vi "GeoData.vi"() -> ()   [LabVIEW 2017] (continued)
VA\tMecklenburg County\tH1\n23915\t51117\tBaskerville\tVA\tMecklenburg County\tH1\n23071\t51119\tHartfield\tVA\tMiddlesex County\tH1\n23169\t51119\tTopping\tVA\tMiddlesex County\tH1\n23070\t51119\tHardyville\tVA\tMiddlesex County\tH1\n23175\t51119\tUrbanna\tVA\tMiddlesex County\tH1\n23176\t51119\tWake\tVA\tMiddlesex County\tH1\n23079\t51119\tJamaica\tVA\tMiddlesex County\tH1\n23031\t51119\tChristchurch\tVA\tMiddlesex County\tH1\n23092\t51119\tLocust hill\tVA\tMiddlesex County\tH1\n23032\t51119\tChurch view\tVA\tMiddlesex County\tH1\n23180\t51119\tWater view\tVA\tMiddlesex County\tH1\n22504\t51119\tLaneview\tVA\tMiddlesex County\tH1\n23043\t51119\tDeltaville\tVA\tMiddlesex County\tH1\n23149\t51119\tSaluda\tVA\tMiddlesex County\tH1\n24068\t51121\tChristiansburg\tVA\tMontgomery County\tH1\n24128\t51121\tNewport\tVA\tMontgomery County\tH1\n24061\t51121\tBlacksburg\tVA\tMontgomery County\tH1\n24063\t51121\tBlacksburg\tVA\tMontgomery County\tH1\n24149\t51121\tRiner\tVA\tMontgomery County\tH1\n24059\t51121\tBent mountain\tVA\tMontgomery County\tH1\n24347\t51121\tHiwassee\tVA\tMontgomery County\tH1\n24111\t51121\tMc coy\tVA\tMontgomery County\tH1\n24087\t51121\tElliston\tVA\tMontgomery County\tH1\n24141\t51121\tRadford\tVA\tMontgomery County\tH1\n24162\t51121\tShawsville\tVA\tMontgomery County\tH1\n24073\t51121\tChristiansburg\tVA\tMontgomery County\tH1\n24070\t51121\tCatawba\tVA\tMontgomery County\tH1\n24062\t51121\tBlacksburg\tVA\tMontgomery County\tH1\n24138\t51121\tPilot\tVA\tMontgomery County\tH1\n24060\t51121\tBlacksburg\tVA\tMontgomery County\tH1\n22920\t51125\tAfton\tVA\tNelson County\tH1\n22938\t51125\tFaber\tVA\tNelson County\tH1\n22967\t51125\tRoseland\tVA\tNelson County\tH1\n22964\t51125\tPiney river\tVA\tNelson County\tH1\n24599\t51125\tWingina\tVA\tNelson County\tH1\n22976\t51125\tTyro\tVA\tNelson County\tH1\n24483\t51125\tVesuvius\tVA\tNelson County\tH1\n22922\t51125\tArrington\tVA\tNelson County\tH1\n22949\t51125\tLovingston\tVA\tNelson County\tH1\n22952\t51125\tLyndhurst\tVA\tNelson County\tH1\n24521\t51125\tAmherst\tVA\tNelson County\tH1\n22971\t51125\tShipman\tVA\tNelson County\tH1\n24562\t51125\tHowardsville\tVA\tNelson County\tH1\n24464\t51125\tMontebello\tVA\tNelson County\tH1\n22958\t51125\tNellysford\tVA\tNelson County\tH1\n24581\t51125\tNorwood\tVA\tNelson County\tH1\n22937\t51125\tEsmont\tVA\tNelson County\tH1\n22969\t51125\tSchuyler\tVA\tNelson County\tH1\n24553\t51125\tGladstone\tVA\tNelson County\tH1\n23140\t51127\tProvidence forge\tVA\tNew Kent County\tH1\n23141\t51127\tQuinton\tVA\tNew Kent County\tH1\n23124\t51127\tNew kent\tVA\tNew Kent County\tH1\n23011\t51127\tBarhamsville\tVA\tNew Kent County\tH1\n23089\t51127\tLanexa\tVA\tNew Kent County\tH1\n23111\t51127\tMechanicsville\tVA\tNew Kent County\tH1\n23181\t51127\tWest point\tVA\tNew Kent County\tH1\n23307\t51131\tBirdsnest\tVA\tNorthampton County\tH1\n23347\t51131\tEastville\tVA\tNorthampton County\tH1\n23316\t51131\tCheriton\tVA\tNorthampton County\tH1\n23354\t51131\tFranktown\tVA\tNorthampton County\tH1\n23350\t51131\tExmore\tVA\tNorthampton County\tH1\n23413\t51131\tNassawadox\tVA\tNorthampton County\tH1\n23429\t51131\tSeaview\tVA\tNorthampton County\tH1\n23443\t51131\tTownsend\tVA\tNorthampton County\tH1\n23408\t51131\tMarionville\tVA\tNorthampton County\tH1\n23313\t51131\tCapeville\tVA\tNorthampton County\tH1\n23405\t51131\tMachipongo\tVA\tNorthampton County\tH1\n23310\t51131\tCape charles\tVA\tNorthampton County\tH1\n23398\t51131\tJamesville\tVA\tNorthampton County\tH1\n23486\t51131\tWillis wharf\tVA\tNorthampton County\tH1\n22460\t51133\tFarnham\tVA\tNorthumberland County\tH1\n22435\t51133\tCallao\tVA\tNorthumberland County\tH1\n22482\t51133\tKilmarnock\tVA\tNorthumberland County\tH1\n22503\t51133\tLancaster\tVA\tNorthumberland County\tH1\n22511\t51133\tLottsburg\tVA\tNorthumberland County\tH1\n22432\t51133\tBurgess\tVA\tNorthumberland County\tH1\n22530\t51133\tOphelia\tVA\tNorthumberland County\tH1\n22579\t51133\tWicomico church\tVA\tNorthumberland County\tH1\n22473\t51133\tHeathsville\tVA\tNorthumberland County\tH1\n22539\t51133\tReedville\tVA\tNorthumberland County\tH1\n23083\t51135\tJetersville\tVA\tNottoway County\tH1\n23922\t51135\tBurkeville\tVA\tNottoway County\tH1\n23966\t51135\tRice\tVA\tNottoway County\tH1\n23002\t51135\tAmelia court house\tVA\tNottoway County\tH1\n23955\t51135\tNottoway\tVA\tNottoway County\tH1\n23824\t51135\tBlackstone\tVA\tNottoway County\tH1\n23894\t51135\tWilsons\tVA\tNottoway County\tH1\n23930\t51135\tCrewe\tVA\tNottoway County\tH1\n23093\t51137\tLouisa\tVA\tOrange County\tH1\n22957\t51137\tMontpelier station\tVA\tOrange County\tH1\n22567\t51137\tUnionville\tVA\tOrange County\tH1\n22551\t51137\tSpotsylvania\tVA\tOrange County\tH1\n22942\t51137\tGordonsville\tVA\tOrange County\tH1\n22972\t51137\tSomerset\tVA\tOrange County\tH1\n22733\t51137\tRapidan\tVA\tOrange County\tH1\n22508\t51137\tLocust grove\tVA\tOrange County\tH1\n22923\t51137\tBarboursville\tVA\tOrange County\tH1\n22701\t51137\tCulpeper\tVA\tOrange County\tH1\n22968\t51137\tRuckersville\tVA\tOrange County\tH1\n22433\t51137\tBurr hill\tVA\tOrange County\tH1\n22542\t51137\tRhoadesville\tVA\tOrange County\tH1\n22960\t51137\tOrange\tVA\tOrange County\tH1\n22827\t51139\tElkton\tVA\tPage County\tH1\n22851\t51139\tStanley\tVA\tPage County\tH1\n22849\t51139\tShenandoah\tVA\tPage County\tH1\n22743\t51139\tSyria\tVA\tPage County\tH1\n22835\t51139\tLuray\tVA\tPage County\tH1\n22650\t51139\tRileyville\tVA\tPage County\tH1\n24133\t51141\tPatrick springs\tVA\tPatrick County\tH1\n24055\t51141\tBassett\tVA\tPatrick County\tH1\n24091\t51141\tFloyd\tVA\tPatrick County\tH1\n24317\t51141\tCana\tVA\tPatrick County\tH1\n24328\t51141\tFancy gap\tVA\tPatrick County\tH1\n24185\t51141\tWoolwine\tVA\tPatrick County\tH1\n24053\t51141\tArarat\tVA\tPatrick County\tH1\n24088\t51141\tFerrum\tVA\tPatrick County\tH1\n24165\t51141\tSpencer\tVA\tPatrick County\tH1\n24343\t51141\tHillsville\tVA\tPatrick County\tH1\n24120\t51141\tMeadows of dan\tVA\tPatrick County\tH1\n24171\t51141\tStuart\tVA\tPatrick County\tH1\n24177\t51141\tVesta\tVA\tPatrick County\tH1\n24076\t51141\tClaudville\tVA\tPatrick County\tH1\n24082\t51141\tCritz\tVA\tPatrick County\tH1\n24380\t51141\tWillis\tVA\tPatrick County\tH1\n24069\t51143\tCascade\tVA\tPittsylvania County\tH1\n24566\t51143\tKeeling\tVA\tPittsylvania County\tH1\n24565\t51143\tJava\tVA\tPittsylvania County\tH1\n24594\t51143\tSutherlin\tVA\tPittsylvania County\tH1\n24139\t51143\tPittsville\tVA\tPittsylvania County\tH1\n24540\t51143\tDanville\tVA\tPittsylvania County\tH1\n24577\t51143\tNathalie\tVA\tPittsylvania County\tH1\n24586\t51143\tRinggold\tVA\tPittsylvania County\tH1\n24054\t51143\tAxton\tVA\tPittsylvania County\tH1\n24527\t51143\tBlairs\tVA\tPittsylvania County\tH1\n24597\t51143\tVernon hill\tVA\tPittsylvania County\tH1\n24563\t51143\tHurt\tVA\tPittsylvania County\tH1\n24161\t51143\tSandy level\tVA\tPittsylvania County\tH1\n24137\t51143\tPenhook\tVA\tPittsylvania County\tH1\n24530\t51143\tCallands\tVA\tPittsylvania County\tH1\n24557\t51143\tGretna\tVA\tPittsylvania County\tH1\n24569\t51143\tLong island\tVA\tPittsylvania County\tH1\n24592\t51143\tSouth boston\tVA\tPittsylvania County\tH1\n24531\t51143\tChatham\tVA\tPittsylvania County\tH1\n24541\t51143\tDanville\tVA\tPittsylvania County\tH1\n24549\t51143\tDry fork\tVA\tPittsylvania County\tH1\n23113\t51145\tMidlothian\tVA\tPowhatan County\tH1\n23112\t51145\tMidlothian\tVA\tPowhatan County\tH1\n23160\t51145\tState farm\tVA\tPowhatan County\tH1\n23120\t51145\tMoseley\tVA\tPowhatan County\tH1\n23139\t51145\tPowhatan\tVA\tPowhatan County\tH1\n23922\t51147\tBurkeville\tVA\tPrince Edward County\tH1\n23966\t51147\tRice\tVA\tPrince Edward County\tH1\n23901\t51147\tFarmville\tVA\tPrince Edward County\tH1\n23947\t51147\tKeysville\tVA\tPrince Edward County\tH1\n23960\t51147\tProspect\tVA\tPrince Edward County\tH1\n23909\t51147\tFarmville\tVA\tPrince Edward County\tH1\n23942\t51147\tGreen bay\tVA\tPrince Edward County\tH1\n23934\t51147\tCullen\tVA\tPrince Edward County\tH1\n23954\t51147\tMeherrin\tVA\tPrince Edward County\tH1\n23943\t51147\tHampden sydney\tVA\tPrince Edward County\tH1\n23923\t51147\tCharlotte court house\tVA\tPrince Edward County\tH1\n23958\t51147\tPamplin\tVA\tPrince Edward County\tH1\n23803\t51149\tPetersburg\tVA\tPrince George County\tH1\n23842\t51149\tDisputanta\tVA\tPrince George County\tH1\n23805\t51149\tPetersburg\tVA\tPrince George County\tH1\n23860\t51149\tHopewell\tVA\tPrince George County\tH1\n23875\t51149\tPrince george\tVA\tPrince George County\tH1\n23881\t51149\tSpring grove\tVA\tPrince George County\tH1\n23801\t51149\tFort lee\tVA\tPrince George County\tH1\n23830\t51149\tCarson\tVA\tPrince George County\tH1\n20155\t51153\tGainesville\tVA\tPrince William County\tH1\n22193\t51153\tWoodbridge\tVA\tPrince William County\tH1\n20109\t51153\tManassas\tVA\tPrince William County\tH1\n20168\t51153\tHaymarket\tVA\tPrince William County\tH1\n20181\t51153\tNokesville\tVA\tPrince William County\tH1\n22026\t51153\tDumfries\tVA\tPrince William County\tH1\n22194\t51153\tWoodbridge\tVA\tPrince William County\tH1\n22192\t51153\tWoodbridge\tVA\tPrince William County\tH1\n20182\t51153\tNokesville\tVA\tPrince William County\tH1\n20111\t51153\tManassas\tVA\tPrince William County\tH1\n20110\t51153\tManassas\tVA\tPrince William County\tH1\n20137\t51153\tBroad run\tVA\tPrince William County\tH1\n22195\t51153\tWoodbridge\tVA\tPrince William County\tH1\n20112\t51153\tManassas\tVA\tPrince William County\tH1\n20169\t51153\tHaymarket\tVA\tPrince William County\tH1\n22025\t51153\tDumfries\tVA\tPrince William County\tH1\n22125\t51153\tOccoquan\tVA\tPrince William County\tH1\n22172\t51153\tTriangle\tVA\tPrince William County\tH1\n22191\t51153\tWoodbridge\tVA\tPrince William County\tH1\n20119\t51153\tCatlett\tVA\tPrince William County\tH1\n20136\t51153\tBristow\tVA\tPrince William County\tH1\n20156\t51153\tGainesville\tVA\tPrince William County\tH1\n22134\t51153\tQuantico\tVA\tPrince William County\tH1\n20143\t51153\tCatharpin\tVA\tPrince William County\tH1\n24084\t51155\tDublin\tVA\tPulaski County\tH1\n24324\t51155\tDraper\tVA\tPulaski County\tH1\n24126\t51155\tNewbern\tVA\tPulaski County\tH1\n24301\t51155\tPulaski\tVA\tPulaski County\tH1\n24347\t51155\tHiwassee\tVA\tPulaski County\tH1\n24141\t51155\tRadford\tVA\tPulaski County\tH1\n24313\t51155\tBarren springs\tVA\tPulaski County\tH1\n24058\t51155\tBelspring\tVA\tPulaski County\tH1\n22630\t51157\tFront royal\tVA\tRappahannock County\tH1\n22640\t51157\tHuntly\tVA\tRappahannock County\tH1\n22747\t51157\tWashington\tVA\tRappahannock County\tH1\n20106\t51157\tAmissville\tVA\tRappahannock County\tH1\n22716\t51157\tCastleton\tVA\tRappahannock County\tH1\n22713\t51157\tBoston\tVA\tRappahannock County\tH1\n22623\t51157\tChester gap\tVA\tRappahannock County\tH1\n22740\t51157\tSperryville\tVA\tRappahannock County\tH1\n22627\t51157\tFlint hill\tVA\tRappahannock County\tH1\n22749\t51157\tWoodville\tVA\tRappahannock County\tH1\n22460\t51159\tFarnham\tVA\tRichmond County\tH1\n22572\t51159\tWarsaw\tVA\tRichmond County\tH1\n22548\t51159\tSharps\tVA\tRichmond County\tH1\n22472\t51159\tHaynesville\tVA\tRichmond County\tH1\n22435\t51159\tCallao\tVA\tRichmond County\tH1\n22503\t51159\tLancaster\tVA\tRichmond County\tH1\n22473\t51159\tHeathsville\tVA\tRichmond County\tH1\n22520\t51159\tMontross\tVA\tRichmond County\tH1\n24014\t51161\tRoanoke\tVA\tRoanoke County\tH1\n24012\t51161\tRoanoke\tVA\tRoanoke County\tH1\n24175\t51161\tTroutville\tVA\tRoanoke County\tH1\n24065\t51161\tBoones mill\tVA\tRoanoke County\tH1\n24153\t51161\tSalem\tVA\tRoanoke County\tH1\n24059\t51161\tBent mountain\tVA\tRoanoke County\tH1\n24079\t51161\tCopper hill\tVA\tRoanoke County\tH1\n24101\t51161\tHardy\tVA\tRoanoke County\tH1\n24179\t51161\tVinton\tVA\tRoanoke County\tH1\n24020\t51161\tRoanoke\tVA\tRoanoke County\tH1\n24087\t51161\tElliston\tVA\tRoanoke County\tH1\n24019\t51161\tRoanoke\tVA\tRoanoke County\tH1\n24070\t51161\tCatawba\tVA\tRoanoke County\tH1\n24018\t51161\tRoanoke\tVA\tRoanoke County\tH1\n24015\t51161\tRoanoke\tVA\tRoanoke County\tH1\n24579\t51163\tNatural bridge station\tVA\tRockbridge County\tH1\n24416\t51163\tBuena vista\tVA\tRockbridge County\tH1\n24066\t51163\tBuchanan\tVA\tRockbridge County\tH1\n24578\t51163\tNatural bridge\tVA\tRockbridge County\tH1\n24435\t51163\tFairfield\tVA\tRockbridge County\tH1\n24450\t51163\tLexington\tVA\tRockbridge County\tH1\n24483\t51163\tVesuvius\tVA\tRockbridge County\tH1\n24472\t51163\tRaphine\tVA\tRockbridge County\tH1\n24459\t51163\tMiddlebrook\tVA\tRockbridge County\tH1\n24555\t51163\tGlasgow\tVA\tRockbridge County\tH1\n24473\t51163\tRockbridge baths\tVA\tRockbridge County\tH1\n24476\t51163\tSteeles tavern\tVA\tRockbridge County\tH1\n24415\t51163\tBrownsburg\tVA\tRockbridge County\tH1\n24439\t51163\tGoshen\tVA\tRockbridge County\tH1\n22801\t51165\tHarrisonburg\tVA\tRockingham County\tH1\n22827\t51165\tElkton\tVA\tRockingham County\tH1\n22840\t51165\tMc gaheysville\tVA\tRockingham County\tH1\n22831\t51165\tHinton\tVA\tRockingham County\tH1\n24471\t51165\tPort republic\tVA\tRockingham County\tH1\n22846\t51165\tPenn laird\tVA\tRockingham County\tH1\n22848\t51165\tPleasant valley\tVA\tRockingham County\tH1\n22833\t51165\tLacey spring\tVA\tRockingham County\tH1\n22821\t51165\tDayton\tVA\tRockingham County\tH1\n22850\t51165\tSingers glen\tVA\tRockingham County\tH1\n22849\t51165\tShenandoah\tVA\tRockingham County\tH1\n22811\t51165\tBergton\tVA\tRockingham County\tH1\n22802\t51165\tHarrisonburg\tVA\tRockingham County\tH1\n22841\t51165\tMount crawford\tVA\tRockingham County\tH1\n24486\t51165\tWeyers cave\tVA\tRockingham County\tH1\n22812\t51165\tBridgewater\tVA\tRockingham County\tH1\n24441\t51165\tGrottoes\tVA\tRockingham County\tH1\n22832\t51165\tKeezletown\tVA\tRockingham County\tH1\n22815\t51165\tBroadway\tVA\tRockingham County\tH1\n22844\t51165\tNew market\tVA\tRockingham County\tH1\n22820\t51165\tCriders\tVA\tRockingham County\tH1\n22834\t51165\tLinville\tVA\tRockingham County\tH1\n22830\t51165\tFulks run\tVA\tRockingham County\tH1\n22853\t51165\tTimberville\tVA\tRockingham County\tH1\n24237\t51167\tDante\tVA\tRussell County\tH1\n24266\t51167\tLebanon\tVA\tRussell County\tH1\n24225\t51167\tCleveland\tVA\tRussell County\tH1\n24283\t51167\tSaint paul\tVA\tRussell County\tH1\n24609\t51167\tCedar bluff\tVA\tRussell County\tH1\n24639\t51167\tRaven\tVA\tRussell County\tH1\n24224\t51167\tCastlewood\tVA\tRussell County\tH1\n24280\t51167\tRosedale\tVA\tRussell County\tH1\n24271\t51167\tNickelsville\tVA\tRussell County\tH1\n24260\t51167\tHonaker\tVA\tRussell County\tH1\n24649\t51167\tSwords creek\tVA\tRussell County\tH1\n24646\t51167\tRowe\tVA\tRussell County\tH1\n24221\t51169\tBlackwater\tVA\tScott County\tH1\n24230\t51169\tCoeburn\tVA\tScott County\tH1\n24245\t51169\tDungannon\tVA\tScott County\tH1\n24250\t51169\tFort blackmore\tVA\tScott County\tH1\n24258\t51169\tHiltons\tVA\tScott County\tH1\n24290\t51169\tWeber city\tVA\tScott County\tH1\n24202\t51169\tBristol\tVA\tScott County\tH1\n24251\t51169\tGate city\tVA\tScott County\tH1\n24271\t51169\tNickelsville\tVA\tScott County\tH1\n24244\t51169\tDuffield\tVA\tScott County\tH1\n22645\t51171\tMiddletown\tVA\tShenandoah County\tH1\n22657\t51171\tStrasburg\tVA\tShenandoah County\tH1\n22626\t51171\tFishers hill\tVA\tShenandoah County\tH1\n22842\t51171\tMount jackson\tVA\tShenandoah County\tH1\n22644\t51171\tMaurertown\tVA\tShenandoah County\tH1\n22652\t51171\tFort valley\tVA\tShenandoah County\tH1\n22810\t51171\tBasye\tVA\tShenandoah County\tH1\n22845\t51171\tOrkney springs\tVA\tShenandoah County\tH1\n22664\t51171\tWoodstock\tVA\tShenandoah County\tH1\n22847\t51171\tQuicksburg\tVA\tShenandoah County\tH1\n22824\t51171\tEdinburg\tVA\tShenandoah County\tH1\n22654\t51171\tStar tannery\tVA\tShenandoah County\tH1\n22815\t51171\tBroadway\tVA\tShenandoah County\tH1\n22844\t51171\tNew market\tVA\tShenandoah County\tH1\n22660\t51171\tToms brook\tVA\tShenandoah County\tH1\n22835\t51171\tLuray\tVA\tShenandoah County\tH1\n22853\t51171\tTimberville\tVA\tShenandoah County\tH1\n22641\t51171\tStrasburg\tVA\tShenandoah County\tH1\n24311\t51173\tAtkins\tVA\tSmyth County\tH1\n24316\t51173\tBroadford\tVA\tSmyth County\tH1\n24375\t51173\tSugar grove\tVA\tSmyth County\tH1\n24651\t51173\tTazewell\tVA\tSmyth County\tH1\n24340\t51173\tGlade spring\tVA\tSmyth County\tH1\n24354\t51173\tMarion\tVA\tSmyth County\tH1\n24318\t51173\tCeres\tVA\tSmyth County\tH1\n24370\t51173\tSaltville\tVA\tSmyth County\tH1\n24368\t51173\tRural retreat\tVA\tSmyth County\tH1\n24378\t51173\tTroutdale\tVA\tSmyth County\tH1\n24236\t51173\tDamascus\tVA\tSmyth County\tH1\n24319\t51173\tChilhowie\tVA\tSmyth County\tH1\n24374\t51173\tSpeedwell\tVA\tSmyth County\tH1\n23867\t51175\tJarratt\tVA\tSouthampton County\tH1\n23878\t51175\tSedley\tVA\tSouthampton County\tH1\n23847\t51175\tEmporia\tVA\tSouthampton County\tH1\n23851\t51175\tFranklin\tVA\tSouthampton County\tH1\n23898\t51175\tZuni\tVA\tSouthampton County\tH1\n23837\t51175\tCourtland\tVA\tSouthampton County\tH1\n23844\t51175\tDrewryville\tVA\tSouthampton County\tH1\n23827\t51175\tBoykins\tVA\tSouthampton County\tH1\n23829\t51175\tCapron\tVA\tSouthampton County\tH1\n23828\t51175\tBranchville\tVA\tSouthampton County\tH1\n23866\t51175\tIvor\tVA\tSouthampton County\tH1\n23874\t51175\tNewsoms\tVA\tSouthampton County\tH1\n23888\t51175\tWakefield\tVA\tSouthampton County\tH1\n22408\t51177\tFredericksburg\tVA\tSpotsylvania County\tH1\n22553\t51177\tSpotsylvania\tVA\tSpotsylvania County\tH1\n22534\t51177\tPartlow\tVA\tSpotsylvania County\tH1\n23117\t51177\tMineral\tVA\tSpotsylvania County\tH1\n22567\t51177\tUnionville\tVA\tSpotsylvania County\tH1\n22551\t51177\tSpotsylvania\tVA\tSpotsylvania County\tH1\n22546\t51177\tRuther glen\tVA\tSpotsylvania County\tH1\n22508\t51177\tLocust grove\tVA\tSpotsylvania County\tH1\n22580\t51177\tWoodford\tVA\tSpotsylvania County\tH1\n22404\t51177\tFredericksburg\tVA\tSpotsylvania County\tH1\n23015\t51177\tBeaverdam\tVA\tSpotsylvania County\tH1\n22401\t51177\tFredericksburg\tVA\tSpotsylvania County\tH1\n22407\t51177\tFredericksburg\tVA\tSpotsylvania County\tH1\n22960\t51177\tOrange\tVA\tSpotsylvania County\tH1\n23024\t51177\tBumpass\tVA\tSpotsylvania County\tH1\n22565\t51177\tThornburg\tVA\tSpotsylvania County\tH1\n22406\t51179\tFredericksburg\tVA\tStafford County\tH1\n22405\t51179\tFredericksburg\tVA\tStafford County\tH1\n22554\t51179\tStafford\tVA\tStafford County\tH1\n22545\t51179\tRuby\tVA\tStafford County\tH1\n22412\t51179\tFredericksburg\tVA\tStafford County\tH1\n22555\t51179\tStafford\tVA\tStafford County\tH1\n22135\t51179\tQuantico\tVA\tStafford County\tH1\n22556\t51179\tStafford\tVA\tStafford County\tH1\n22403\t51179\tFredericksburg\tVA\tStafford County\tH1\n22430\t51179\tBrooke\tVA\tStafford County\tH1\n22471\t51179\tHartwood\tVA\tStafford County\tH1\n22728\t51179\tMidland\tVA\tStafford County\tH1\n22463\t51179\tGarrisonville\tVA\tStafford County\tH1\n22134\t51179\tQuantico\tVA\tStafford County\tH1\n23846\t51181\tElberon\tVA\tSurry County\tH1\n23890\t51181\tWaverly\tVA\tSurry County\tH1\n23899\t51181\tClaremont\tVA\tSurry County\tH1\n23842\t51181\tDisputanta\tVA\tSurry County\tH1\n23883\t51181\tSurry\tVA\tSurry County\tH1\n23839\t51181\tDendron\tVA\tSurry County\tH1\n23430\t51181\tSmithfield\tVA\tSurry County\tH1\n23881\t51181\tSpring grove\tVA\tSurry County\tH1\n23866\t51181\tIvor\tVA\tSurry County\tH1\n23888\t51181\tWakefield\tVA\tSurry County\tH1\n23867\t51183\tJarratt\tVA\tSussex County\tH1\n23878\t51183\tSedley\tVA\tSussex County\tH1\n23890\t51183\tWaverly\tVA\tSussex County\tH1\n23847\t51183\tEmporia\tVA\tSussex County\tH1\n23842\t51183\tDisputanta\tVA\tSussex County\tH1\n23891\t51183\tWaverly\tVA\tSussex County\tH1\n23897\t51183\tYale\tVA\tSussex County\tH1\n23837\t51183\tCourtland\tVA\tSussex County\tH1\n23829\t51183\tCapron\tVA\tSussex County\tH1\n23882\t51183\tStony creek\tVA\tSussex County\tH1\n23830\t51183\tCarson\tVA\tSussex County\tH1\n23888\t51183\tWakefield\tVA\tSussex County\tH1\n23884\t51183\tSussex\tVA\tSussex County\tH1\n24630\t51185\tNorth tazewell\tVA\tTazewell County\tH1\n24316\t51185\tBroadford\tVA\tTazewell County\tH1\n24604\t51185\tBishop\tVA\tTazewell County\tH1\n24314\t51185\tBastian\tVA\tTazewell County\tH1\n24651\t51185\tTazewell\tVA\tTazewell County\tH1\n24602\t51185\tBandy\tVA\tTazewell County\tH1\n24622\t51185\tJewell ridge\tVA\tTazewell County\tH1\n24612\t51185\tDoran\tVA\tTazewell County\tH1\n24647\t51185\tShortt gap\tVA\tTazewell County\tH1\n24377\t51185\tTannersville\tVA\tTazewell County\tH1\n24609\t51185\tCedar bluff\tVA\tTazewell County\tH1\n24606\t51185\tBoissevain\tVA\tTazewell County\tH1\n24640\t51185\tRed ash\tVA\tTazewell County\tH1\n24641\t51185\tRichlands\tVA\tTazewell County\tH1\n24619\t51185\tHorsepen\tVA\tTazewell County\tH1\n24639\t51185\tRaven\tVA\tTazewell County\tH1\n24635\t51185\tPocahontas\tVA\tTazewell County\tH1\n24608\t51185\tBurkes garden\tVA\tTazewell County\tH1\n24605\t51185\tBluefield\tVA\tTazewell County\tH1\n24637\t51185\tPounding mill\tVA\tTazewell County\tH1\n24601\t51185\tAmonate\tVA\tTazewell County\tH1\n24613\t51185\tFalls mills\tVA\tTazewell County\tH1\n22630\t51187\tFront royal\tVA\tWarren County\tH1\n22645\t51187\tMiddletown\tVA\tWarren County\tH1\n22649\t51187\tMiddletown\tVA\tWarren County\tH1\n22657\t51187\tStrasburg\tVA\tWarren County\tH1\n22623\t51187\tChester gap\tVA\tWarren County\tH1\n22642\t51187\tLinden\tVA\tWarren County\tH1\n22610\t51187\tBentonville\tVA\tWarren County\tH1\n22655\t51187\tStephens city\tVA\tWarren County\tH1\n22663\t51187\tWhite post\tVA\tWarren County\tH1\n24212\t51191\tAbingdon\tVA\tWashington County\tH1\n24361\t51191\tMeadowview\tVA\tWashington County\tH1\n24327\t51191\tEmory\tVA\tWashington County\tH1\n24340\t51191\tGlade spring\tVA\tWashington County\tH1\n24258\t51191\tHiltons\tVA\tWashington County\tH1\n24370\t51191\tSaltville\tVA\tWashington County\tH1\n24211\t51191\tAbingdon\tVA\tWashington County\tH1\n24270\t51191\tMendota\tVA\tWashington County\tH1\n24202\t51191\tBristol\tVA\tWashington County\tH1\n24210\t51191\tAbingdon\tVA\tWashington County\tH1\n24292\t51191\tWhitetop\tVA\tWashington County\tH1\n24236\t51191\tDamascus\tVA\tWashington County\tH1\n24319\t51191\tChilhowie\tVA\tWashington County\tH1\n22572\t51193\tWarsaw\tVA\tWestmoreland County\tH1\n22529\t51193\tOldhams\tVA\tWestmoreland County\tH1\n22435\t51193\tCallao\tVA\tWestmoreland County\tH1\n22442\t51193\tColes point\tVA\tWestmoreland County\tH1\n22581\t51193\tZacata\tVA\tWestmoreland County\tH1\n22524\t51193\tMount holly\tVA\tWestmoreland County\tH1\n22558\t51193\tStratford\tVA\tWestmoreland County\tH1\n22443\t51193\tColonial beach\tVA\tWestmoreland County\tH1\n22469\t51193\tHague\tVA\tWestmoreland County\tH1\n22485\t51193\tKing george\tVA\tWestmoreland County\tH1\n22488\t51193\tKinsale\tVA\tWestmoreland County\tH1\n22577\t51193\tSandy point\tVA\tWestmoreland County\tH1\n22520\t51193\tMontross\tVA\tWestmoreland County\tH1\n24219\t51195\tBig stone gap\tVA\tWise County\tH1\n24230\t51195\tCoeburn\tVA\tWise County\tH1\n24283\t51195\tSaint paul\tVA\tWise County\tH1\n24293\t51195\tWise\tVA\tWise County\tH1\n24246\t51195\tEast stone gap\tVA\tWise County\tH1\n24273\t51195\tNorton\tVA\tWise County\tH1\n24279\t51195\tPound\tVA\tWise County\tH1\n24215\t51195\tAndover\tVA\tWise County\tH1\n24216\t51195\tAppalachia\tVA\tWise County\tH1\n24324\t51197\tDraper\tVA\tWythe County\tH1\n24360\t51197\tMax meadows\tVA\tWythe County\tH1\n24322\t51197\tCripple creek\tVA\tWythe County\tH1\n24350\t51197\tIvanhoe\tVA\tWythe County\tH1\n24343\t51197\tHillsville\tVA\tWythe County\tH1\n24368\t51197\tRural retreat\tVA\tWythe County\tH1\n24313\t51197\tBarren springs\tVA\tWythe County\tH1\n24312\t51197\tAustinville\tVA\tWythe County\tH1\n24382\t51197\tWytheville\tVA\tWythe County\tH1\n24323\t51197\tCrockett\tVA\tWythe County\tH1\n24374\t51197\tSpeedwell\tVA\tWythe County\tH1\n23185\t51199\tWilliamsburg\tVA\tYork County\tH1\n23602\t51199\tNewport news\tVA\tYork County\tH1\n23692\t51199\tYorktown\tVA\tYork County\tH1\n23696\t51199\tSeaford\tVA\tYork County\tH1\n23188\t51199\tWilliamsburg\tVA\tYork County\tH1\n23691\t51199\tYorktown\tVA\tYork County\tH1\n23693\t51199\tYorktown\tVA\tYork County\tH1\n23603\t51199\tNewport news\tVA\tYork County\tH1\n23690\t51199\tYorktown\tVA\tYork County\tH1\n23665\t51199\tHampton\tVA\tYork County\tH1\n23694\t51199\tLackey\tVA\tYork County\tH1\n23090\t51199\tLightfoot\tVA\tYork County\tH1\n22305\t51510\tAlexandria\tVA\tAlexandria city\tC7\n22350\t51510\tAlexandria\tVA\tAlexandria city\tC7\n22320\t51510\tAlexandria\tVA\tAlexandria city\tC7\n22312\t51510\tAlexandria\tVA\tAlexandria city\tC7\n22332\t51510\tAlexandria\tVA\tAlexandria city\tC7\n22333\t51510\tAlexandria\tVA\tAlexandria city\tC7\n22302\t51510\tAlexandria\tVA\tAlexandria city\tC7\n22304\t51510\tAlexandria\tVA\tAlexandria city\tC7\n22314\t51510\tAlexandria\tVA\tAlexandria city\tC7\n22313\t51510\tAlexandria\tVA\tAlexandria city\tC7\n20598\t51510\tDhs\tVA\tAlexandria city\tC7\n22301\t51510\tAlexandria\tVA\tAlexandria city\tC7\n22331\t51510\tAlexandria\tVA\tAlexandria city\tC7\n22206\t51510\tArlington\tVA\tAlexandria city\tC7\n22311\t51510\tAlexandria\tVA\tAlexandria city\tC7\n24203\t51520\tBristol\tVA\tBristol city\tC7\n24201\t51520\tBristol\tVA\tBristol city\tC7\n24202\t51520\tBristol\tVA\tBristol city\tC7\n24209\t51520\tBristol\tVA\tBristol city\tC7\n24416\t51530\tBuena vista\tVA\tBuena Vista city\tC7\n22903\t51540\tCharlottesville\tVA\tCharlottesville city\tC7\n22901\t51540\tCharlottesville\tVA\tCharlottesville city\tC7\n22902\t51540\tCharlottesville\tVA\tCharlottesville city\tC7\n22906\t51540\tCharlottesville\tVA\tCharlottesville city\tC7\n22908\t51540\tCharlottesville\tVA\tCharlottesville city\tC7\n22905\t51540\tCharlottesville\tVA\tCharlottesville city\tC7\n23323\t51550\tChesapeake\tVA\tChesapeake city\tC7\n23326\t51550\tChesapeake\tVA\tChesapeake city\tC7\n23322\t51550\tChesapeake\tVA\tChesapeake city\tC7\n23320\t51550\tChesapeake\tVA\tChesapeake city\tC7\n23321\t51550\tChesapeake\tVA\tChesapeake city\tC7\n23324\t51550\tChesapeake\tVA\tChesapeake city\tC7\n23703\t51550\tPortsmouth\tVA\tChesapeake city\tC7\n23328\t51550\tChesapeake\tVA\tChesapeake city\tC7\n23325\t51550\tChesapeake\tVA\tChesapeake city\tC7\n23435\t51550\tSuffolk\tVA\tChesapeake city\tC7\n23702\t51550\tPortsmouth\tVA\tChesapeake city\tC7\n23327\t51550\tChesapeake\tVA\tChesapeake city\tC7\n23464\t51550\tVirginia beach\tVA\tChesapeake city\tC7\n23834\t51570\tColonial heights\tVA\tColonial Heights city\tC7\n24426\t51580\tCovington\tVA\tCovington city\tC7\n24540\t51590\tDanville\tVA\tDanville city\tC7\n24541\t51590\tDanville\tVA\tDanville city\tC7\n23847\t51595\tEmporia\tVA\tEmporia city\tC7\n22030\t51600\tFairfax\tVA\tFairfax city\tC7\n22038\t51600\tFairfax\tVA\tFairfax city\tC7\n22031\t51600\tFairfax\tVA\tFairfax city\tC7\n22032\t51600\tFairfax\tVA\tFairfax city\tC7\n22205\t51610\tArlington\tVA\tFalls Church city\tC7\n22044\t51610\tFalls church\tVA\tFalls Church city\tC7\n22046\t51610\tFalls church\tVA\tFalls Church city\tC7\n22213\t51610\tArlington\tVA\tFalls Church city\tC7\n22042\t51610\tFalls church\tVA\tFalls Church city\tC7\n22040\t51610\tFalls church\tVA\tFalls Church city\tC7\n23851\t51620\tFranklin\tVA\tFranklin city\tC7\n22408\t51630\tFredericksburg\tVA\tFredericksburg city\tC7\n22402\t51630\tFredericksburg\tVA\tFredericksburg city\tC7\n22404\t51630\tFredericksburg\tVA\tFredericksburg city\tC7\n22401\t51630\tFredericksburg\tVA\tFredericksburg city\tC7\n22407\t51630\tFredericksburg\tVA\tFredericksburg city\tC7\n24333\t51640\tGalax\tVA\tGalax city\tC7\n23607\t51650\tNewport news\tVA\tHampton city\tC7\n23670\t51650\tHampton\tVA\tHampton city\tC7\n23663\t51650\tHampton\tVA\tHampton city\tC7\n23669\t51650\tHampton\tVA\tHampton city\tC7\n23662\t51650\tPoquoson\tVA\tHampton city\tC7\n23651\t51650\tFort monroe\tVA\tHampton city\tC7\n23666\t51650\tHampton\tVA\tHampton city\tC7\n23668\t51650\tHampton\tVA\tHampton city\tC7\n23630\t51650\tHampton\tVA\tHampton city\tC7\n23661\t51650\tHampton\tVA\tHampton city\tC7\n23665\t51650\tHampton\tVA\tHampton city\tC7\n23605\t51650\tNewport news\tVA\tHampton city\tC7\n23681\t51650\tHampton\tVA\tHampton city\tC7\n23664\t51650\tHampton\tVA\tHampton city\tC7\n23667\t51650\tHampton\tVA\tHampton city\tC7\n22801\t51660\tHarrisonburg\tVA\tHarrisonburg city\tC7\n22802\t51660\tHarrisonburg\tVA\tHarrisonburg city\tC7\n22803\t51660\tHarrisonburg\tVA\tHarrisonburg city\tC7\n22807\t51660\tHarrisonburg\tVA\tHarrisonburg city\tC7\n23860\t51670\tHopewell\tVA\tHopewell city\tC7\n24450\t51678\tLexington\tVA\tLexington city\tC7\n24515\t51680\tLynchburg\tVA\tLynchburg city\tC7\n24504\t51680\tLynchburg\tVA\tLynchburg city\tC7\n24503\t51680\tLynchburg\tVA\tLynchburg city\tC7\n24506\t51680\tLynchburg\tVA\tLynchburg city\tC7\n24513\t51680\tLynchburg\tVA\tLynchburg city\tC7\n24502\t51680\tLynchburg\tVA\tLynchburg city\tC7\n24514\t51680\tLynchburg\tVA\tLynchburg city\tC7\n24501\t51680\tLynchburg\tVA\tLynchburg city\tC7\n24551\t51680\tForest\tVA\tLynchburg city\tC7\n20110\t51683\tManassas\tVA\tManassas city\tC7\n20108\t51683\tManassas\tVA\tManassas city\tC7\n20111\t51685\tManassas\tVA\tManassas Park city\tC7\n20110\t51685\tManassas\tVA\tManassas Park city\tC7\n20113\t51685\tManassas\tVA\tManassas Park city\tC7\n24112\t51690\tMartinsville\tVA\tMartinsville city\tC7\n23606\t51700\tNewport news\tVA\tNewport News city\tC7\n23601\t51700\tNewport news\tVA\tNewport News city\tC7\n23602\t51700\tNewport news\tVA\tNewport News city\tC7\n23607\t51700\tNewport news\tVA\tNewport News city\tC7\n23609\t51700\tNewport news\tVA\tNewport News city\tC7\n23670\t51700\tHampton\tVA\tNewport News city\tC7\n23604\t51700\tFort eustis\tVA\tNewport News city\tC7\n23612\t51700\tNewport news\tVA\tNewport News city\tC7\n23608\t51700\tNewport news\tVA\tNewport News city\tC7\n23666\t51700\tHampton\tVA\tNewport News city\tC7\n23630\t51700\tHampton\tVA\tNewport News city\tC7\n23603\t51700\tNewport news\tVA\tNewport News city\tC7\n23690\t51700\tYorktown\tVA\tNewport News city\tC7\n23605\t51700\tNewport news\tVA\tNewport News city\tC7\n23628\t51700\tNewport news\tVA\tNewport News city\tC7\n23505\t51710\tNorfolk\tVA\tNorfolk city\tC7\n23510\t51710\tNorfolk\tVA\tNorfolk city\tC7\n23551\t51710\tNorfolk\tVA\tNorfolk city\tC7\n23503\t51710\tNorfolk\tVA\tNorfolk city\tC7\n23509\t51710\tNorfolk\tVA\tNorfolk city\tC7\n23513\t51710\tNorfolk\tVA\tNorfolk city\tC7\n23529\t51710\tNorfolk\tVA\tNorfolk city\tC7\n23462\t51710\tVirginia beach\tVA\tNorfolk city\tC7\n23518\t51710\tNorfolk\tVA\tNorfolk city\tC7\n23523\t51710\tNorfolk\tVA\tNorfolk city\tC7\n23502\t51710\tNorfolk\tVA\tNorfolk city\tC7\n23511\t51710\tNorfolk\tVA\tNorfolk city\tC7\n23517\t51710\tNorfolk\tVA\tNorfolk city\tC7\n23514\t51710\tNorfolk\tVA\tNorfolk city\tC7\n23504\t51710\tNorfolk\tVA\tNorfolk city\tC7\n23515\t51710\tNorfolk\tVA\tNorfolk city\tC7\n23507\t51710\tNorfolk\tVA\tNorfolk city\tC7\n23501\t51710\tNorfolk\tVA\tNorfolk city\tC7\n23541\t51710\tNorfolk\tVA\tNorfolk city\tC7\n23508\t51710\tNorfolk\tVA\tNorfolk city\tC7\n24273\t51720\tNorton\tVA\tNorton city\tC7\n23803\t51730\tPetersburg\tVA\tPetersburg city\tC7\n23805\t51730\tPetersburg\tVA\tPetersburg city\tC7\n23875\t51730\tPrince george\tVA\tPetersburg city\tC7\n23801\t51730\tFort lee\tVA\tPetersburg city\tC7\n23804\t51730\tPetersburg\tVA\tPetersburg city\tC7\n23662\t51735\tPoquoson\tVA\tPoquoson city\tC7\n23708\t51740\tPortsmouth\tVA\tPortsmouth city\tC7\n23705\t51740\tPortsmouth\tVA\tPortsmouth city\tC7\n23709\t51740\tPortsmouth\tVA\tPortsmouth city\tC7\n23321\t51740\tChesapeake\tVA\tPortsmouth city\tC7\n23704\t51740\tPortsmouth\tVA\tPortsmouth city\tC7\n23703\t51740\tPortsmouth\tVA\tPortsmouth city\tC7\n23701\t51740\tPortsmouth\tVA\tPortsmouth city\tC7\n23707\t51740\tPortsmouth\tVA\tPortsmouth city\tC7\n23702\t51740\tPortsmouth\tVA\tPortsmouth city\tC7\n24129\t51750\tNew river\tVA\tRadford city\tC7\n24141\t51750\tRadford\tVA\tRadford city\tC7\n24073\t51750\tChristiansburg\tVA\tRadford city\tC7\n24142\t51750\tRadford\tVA\tRadford city\tC7\n24132\t51750\tParrott\tVA\tRadford city\tC7\n23222\t51760\tRichmond\tVA\tRichmond city\tC7\n23221\t51760\tRichmond\tVA\tRichmond city\tC7\n23224\t51760\tRichmond\tVA\tRichmond city\tC7\n23235\t51760\tRichmond\tVA\tRichmond city\tC7\n23218\t51760\tRichmond\tVA\tRichmond city\tC7\n23249\t51760\tRichmond\tVA\tRichmond city\tC7\n23113\t51760\tMidlothian\tVA\tRichmond city\tC7\n23219\t51760\tRichmond\tVA\tRichmond city\tC7\n23231\t51760\tHenrico\tVA\tRichmond city\tC7\n23293\t51760\tRichmond\tVA\tRichmond city\tC7\n23269\t51760\tRichmond\tVA\tRichmond city\tC7\n23220\t51760\tRichmond\tVA\tRichmond city\tC7\n23284\t51760\tRichmond\tVA\tRichmond city\tC7\n23298\t51760\tRichmond\tVA\tRichmond city\tC7\n23241\t51760\tRichmond\tVA\tRichmond city\tC7\n23227\t51760\tRichmond\tVA\tRichmond city\tC7\n23260\t51760\tRichmond\tVA\tRichmond city\tC7\n23223\t51760\tRichmond\tVA\tRichmond city\tC7\n23261\t51760\tRichmond\tVA\tRichmond city\tC7\n23173\t51760\tRichmond\tVA\tRichmond city\tC7\n23226\t51760\tRichmond\tVA\tRichmond city\tC7\n23286\t51760\tRichmond\tVA\tRichmond city\tC7\n23228\t51760\tHenrico\tVA\tRichmond city\tC7\n23230\t51760\tRichmond\tVA\tRichmond city\tC7\n23234\t51760\tRichmond\tVA\tRichmond city\tC7\n23232\t51760\tRichmond\tVA\tRichmond city\tC7\n23225\t51760\tRichmond\tVA\tRichmond city\tC7\n24014\t51770\tRoanoke\tVA\tRoanoke city\tC7\n24012\t51770\tRoanoke\tVA\tRoanoke city\tC7\n24026\t51770\tRoanoke\tVA\tRoanoke city\tC7\n24035\t51770\tRoanoke\tVA\tRoanoke city\tC7\n24036\t51770\tRoanoke\tVA\tRoanoke city\tC7\n24030\t51770\tRoanoke\tVA\tRoanoke city\tC7\n24001\t51770\tRoanoke\tVA\tRoanoke city\tC7\n24042\t51770\tRoanoke\tVA\tRoanoke city\tC7\n24011\t51770\tRoanoke\tVA\tRoanoke city\tC7\n24022\t51770\tRoanoke\tVA\tRoanoke city\tC7\n24153\t51770\tSalem\tVA\tRoanoke city\tC7\n24010\t51770\tRoanoke\tVA\tRoanoke city\tC7\n24031\t51770\tRoanoke\tVA\tRoanoke city\tC7\n24009\t51770\tRoanoke\tVA\tRoanoke city\tC7\n24028\t51770\tRoanoke\tVA\tRoanoke city\tC7\n24034\t51770\tRoanoke\tVA\tRoanoke city\tC7\n24179\t51770\tVinton\tVA\tRoanoke city\tC7\n24027\t51770\tRoanoke\tVA\tRoanoke city\tC7\n24023\t51770\tRoanoke\tVA\tRoanoke city\tC7\n24013\t51770\tRoanoke\tVA\tRoanoke city\tC7\n24006\t51770\tRoanoke\tVA\tRoanoke city\tC7\n24007\t51770\tRoanoke\tVA\tRoanoke city\tC7\n24037\t51770\tRoanoke\tVA\tRoanoke city\tC7\n24016\t51770\tRoanoke\tVA\tRoanoke city\tC7\n24017\t51770\tRoanoke\tVA\tRoanoke city\tC7\n24032\t51770\tRoanoke\tVA\tRoanoke city\tC7\n24008\t51770\tRoanoke\tVA\tRoanoke city\tC7\n24003\t51770\tRoanoke\tVA\tRoanoke city\tC7\n24019\t51770\tRoanoke\tVA\tRoanoke city\tC7\n24005\t51770\tRoanoke\tVA\tRoanoke city\tC7\n24004\t51770\tRoanoke\tVA\tRoanoke city\tC7\n24025\t51770\tRoanoke\tVA\tRoanoke city\tC7\n24024\t51770\tRoanoke\tVA\tRoanoke city\tC7\n24018\t51770\tRoanoke\tVA\tRoanoke city\tC7\n24015\t51770\tRoanoke\tVA\tRoanoke city\tC7\n24038\t51770\tRoanoke\tVA\tRoanoke city\tC7\n24002\t51770\tRoanoke\tVA\tRoanoke city\tC7\n24033\t51770\tRoanoke\tVA\tRoanoke city\tC7\n24029\t51770\tRoanoke\tVA\tRoanoke city\tC7\n24153\t51775\tSalem\tVA\tSalem city\tC7\n24017\t51775\tRoanoke\tVA\tSalem city\tC7\n24019\t51775\tRoanoke\tVA\tSalem city\tC7\n24018\t51775\tRoanoke\tVA\tSalem city\tC7\n24402\t51790\tStaunton\tVA\tStaunton city\tC7\n24482\t51790\tVerona\tVA\tStaunton city\tC7\n24401\t51790\tStaunton\tVA\tStaunton city\tC7\n23432\t51800\tSuffolk\tVA\tSuffolk city\tC7\n23439\t51800\tSuffolk\tVA\tSuffolk city\tC7\n23434\t51800\tSuffolk\tVA\tSuffolk city\tC7\n23438\t51800\tSuffolk\tVA\tSuffolk city\tC7\n23321\t51800\tChesapeake\tVA\tSuffolk city\tC7\n23487\t51800\tWindsor\tVA\tSuffolk city\tC7\n23437\t51800\tSuffolk\tVA\tSuffolk city\tC7\n23430\t51800\tSmithfield\tVA\tSuffolk city\tC7\n23436\t51800\tSuffolk\tVA\tSuffolk city\tC7\n23435\t51800\tSuffolk\tVA\tSuffolk city\tC7\n23433\t51800\tSuffolk\tVA\tSuffolk city\tC7\n23453\t51810\tVirginia beach\tVA\tVirginia Beach city\tC7\n23459\t51810\tVirginia beach\tVA\tVirginia Beach city\tC7\n23479\t51810\tVirginia beach\tVA\tVirginia Beach city\tC7\n23322\t51810\tChesapeake\tVA\tVirginia Beach city\tC7\n23320\t51810\tChesapeake\tVA\tVirginia Beach city\tC7\n23456\t51810\tVirginia beach\tVA\tVirginia Beach city\tC7\n23471\t51810\tVirginia beach\tVA\tVirginia Beach city\tC7\n23454\t51810\tVirginia beach\tVA\tVirginia Beach city\tC7\n23450\t51810\tVirginia beach\tVA\tVirginia Beach city\tC7\n23452\t51810\tVirginia beach\tVA\tVirginia Beach city\tC7\n23462\t51810\tVirginia beach\tVA\tVirginia Beach city\tC7\n23466\t51810\tVirginia beach\tVA\tVirginia Beach city\tC7\n23460\t51810\tVirginia beach\tVA\tVirginia Beach city\tC7\n23461\t51810\tVirginia beach\tVA\tVirginia Beach city\tC7\n23325\t51810\tChesapeake\tVA\tVirginia Beach city\tC7\n23502\t51810\tNorfolk\tVA\tVirginia Beach city\tC7\n23463\t51810\tVirginia beach\tVA\tVirginia Beach city\tC7\n23455\t51810\tVirginia beach\tVA\tVirginia Beach city\tC7\n23467\t51810\tVirginia beach\tVA\tVirginia Beach city\tC7\n23451\t51810\tVirginia beach\tVA\tVirginia Beach city\tC7\n23464\t51810\tVirginia beach\tVA\tVirginia Beach city\tC7\n23457\t51810\tVirginia beach\tVA\tVirginia Beach city\tC7\n22980\t51820\tWaynesboro\tVA\tWaynesboro city\tC7\n22952\t51820\tLyndhurst\tVA\tWaynesboro city\tC7\n23185\t51830\tWilliamsburg\tVA\tWilliamsburg city\tC7\n23188\t51830\tWilliamsburg\tVA\tWilliamsburg city\tC7\n23186\t51830\tWilliamsburg\tVA\tWilliamsburg city\tC7\n23187\t51830\tWilliamsburg\tVA\tWilliamsburg city\tC7\n22601\t51840\tWinchester\tVA\tWinchester city\tC7\n22602\t51840\tWinchester\tVA\tWinchester city\tC7\n22604\t51840\tWinchester\tVA\tWinchester city\tC7\n98857\t53001\tWarden\tWA\tAdams County\tH1\n99032\t53001\tSprague\tWA\tAdams County\tH1\n99125\t53001\tEndicott\tWA\tAdams County\tH1\n99341\t53001\tLind\tWA\tAdams County\tH1\n99371\t53001\tWashtucna\tWA\tAdams County\tH1\n99169\t53001\tRitzville\tWA\tAdams County\tH1\n99344\t53001\tOthello\tWA\tAdams County\tH1\n99105\t53001\tBenge\tWA\tAdams County\tH1\n98832\t53001\tMarlin\tWA\tAdams County\tH1\n99017\t53001\tLamont\tWA\tAdams County\tH1\n99326\t53001\tConnell\tWA\tAdams County\tH1\n99159\t53001\tOdessa\tWA\tAdams County\tH1\n99402\t53003\tAsotin\tWA\tAsotin County\tH1\n99401\t53003\tAnatone\tWA\tAsotin County\tH1\n99403\t53003\tClarkston\tWA\tAsotin County\tH1\n99354\t53005\tRichland\tWA\tBenton County\tH1\n99352\t53005\tRichland\tWA\tBenton County\tH1\n99338\t53005\tKennewick\tWA\tBenton County\tH1\n99346\t53005\tPlymouth\tWA\tBenton County\tH1\n99336\t53005\tKennewick\tWA\tBenton County\tH1\n99353\t53005\tWest richland\tWA\tBenton County\tH1\n98944\t53005\tSunnyside\tWA\tBenton County\tH1\n99350\t53005\tProsser\tWA\tBenton County\tH1\n99345\t53005\tPaterson\tWA\tBenton County\tH1\n98930\t53005\tGrandview\tWA\tBenton County\tH1\n99320\t53005\tBenton city\tWA\tBenton County\tH1\n99337\t53005\tKennewick\tWA\tBenton County\tH1\n98828\t53007\tMalaga\tWA\tChelan County\tH1\n98816\t53007\tChelan\tWA\tChelan County\tH1\n98822\t53007\tEntiat\tWA\tChelan County\tH1\n98846\t53007\tPateros\tWA\tChelan County\tH1\n98836\t53007\tMonitor\tWA\tChelan County\tH1\n98815\t53007\tCashmere\tWA\tChelan County\tH1\n98817\t53007\tChelan falls\tWA\tChelan County\tH1\n98801\t53007\tWenatchee\tWA\tChelan County\tH1\n98802\t53007\tEast wenatchee\tWA\tChelan County\tH1\n98807\t53007\tWenatchee\tWA\tChelan County\tH1\n98811\t53007\tArdenvoir\tWA\tChelan County\tH1\n98831\t53007\tManson\tWA\tChelan County\tH1\n98852\t53007\tStehekin\tWA\tChelan County\tH1\n98847\t53007\tPeshastin\tWA\tChelan County\tH1\n98826\t53007\tLeavenworth\tWA\tChelan County\tH1\n98821\t53007\tDryden\tWA\tChelan County\tH1\n98381\t53009\tSekiu\tWA\tClallam County\tH1\n98305\t53009\tBeaver\tWA\tClallam County\tH1\n98363\t53009\tPort angeles\tWA\tClallam County\tH1\n98324\t53009\tCarlsborg\tWA\tClallam County\tH1\n98326\t53009\tClallam bay\tWA\tClallam County\tH1\n98382\t53009\tSequim\tWA\tClallam County\tH1\n
